vi "Get Debug Attribute.vi"(8 "error in (no error)":errorcluster, 11 "SMO":refnum<class "SMO.lvclass">) -> (0 "error out":errorcluster, 3 "Attribute.Debug":refnum<class "Attribute.Debug.lvclass">)   [LabVIEW 2019, in "SMO Debug.lvlib" / "SMO.Mediator.lvclass"]
uses:
  SMO.Mediator.lvclass
  <vilib>/JKI/JKI SMO/SMO/SMO.lvclass
  Attribute.Debug/Attribute.Debug.lvclass
  C:/Program Files (x86)/National Instruments/LabVIEW 2019/vi.lib/JKI/JKI SMO/Support/Attribute/Attribute.lvclass
  <vilib>/JKI/JKI SMO/Support/Attribute/Attribute.lvclass/Attribute.ctl
  <vilib>/Utility/LVClass/Get LV Class Name.vi
  <vilib>/JKI/JKI SMO/Support/Attribute/Attribute.lvclass
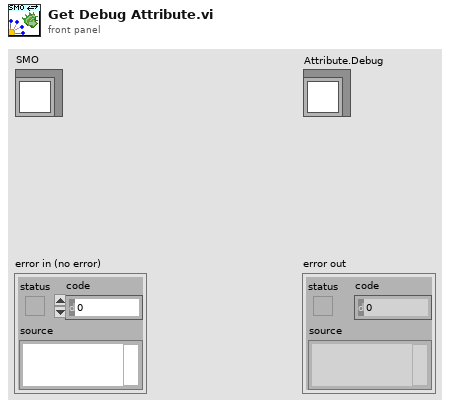
[diagram p1: front panel]
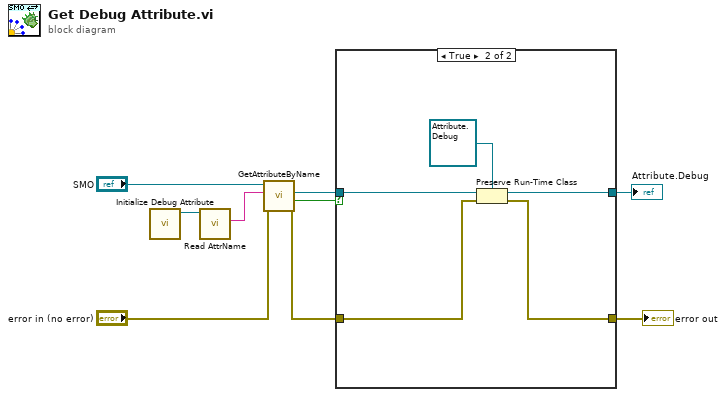
[diagram p0: block diagram]
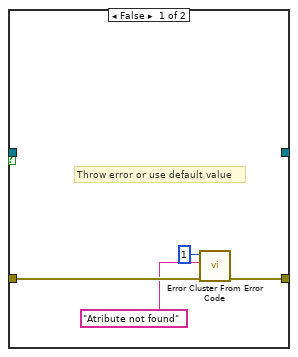
[diagram p2: hidden frame]
diagram:
  n1 = call "Initialize Debug Attribute.vi"() -> ("Attribute.StartupBehavior"=w2:refnum<class "Attribute.Debug.lvclass">)  [unwired: 11 in]
  n2 = call <vilib>:"Read AttrName.vi"("Attribute in"=w2) -> ("Attribute Name"=w1:string)  [unwired: 8 in, 2 out]
  n3 = call <vilib>:"GetAttributeByName.vi"("error in (no error)"="error in (no error)", "AttrName"=w1, "SMO in"="SMO") -> ("error out"=w3:errorcluster, "found"=w6:bool, "Attribute"=w8:refnum<class "Attribute.lvclass">)  [unwired: 5 in, 1 out]
  n4 = case shown="True" w6 {
    tunnel: w8 -> [_ w18]
    tunnel: [_ w16] -> w7
    tunnel: [w13 w15] -> w4
    tunnel: w3 -> [w12 w14]
    frame False {
      # "Throw error or use default value"
      n5 = call <vilib>:"Error Cluster From Error Code.vi"("error in (no error)"=w12, "error message (\"\")"="Atribute not found" ("error message (\"\")"), "error code (0)"=1) -> ("error out"=w13:errorcluster)  [unwired: 6 in]
    }
    frame True {
      n6 = Preserve Run-Time Class(object in=w18, error in=w14, 2:refnum<class "Attribute.Debug.lvclass"> refnum ("SMO Debug.lvlib:Attribute.Debug.lvclass")) -> (object out=w16:refnum<class "Attribute.Debug.lvclass">, error out=w15:errorcluster)
    }
  }
  "error out" <- w4
  "Attribute.Debug" <- w7
